vi "ReadEncoders.vi"(0 "Reset Encoders":bool, 5 "Cluster in":T1={FALSE, "Tick Count(uSec)"=0, "Counter Value"=[0, 0, 0, 0], "x-y"=[0, 0, 0, 0]}, 11 "error in (no error)":errorcluster) -> (4 "Tick Count(uSec)":u32 caption="Tick Count(Ticks)", 8 "output cluster":T2, 13 "Cluster Out":T1, 14 "Updated":bool, 15 "error out":errorcluster)   [LabVIEW 2018]
uses:
  <vilib>/myRIO/Common/Instrument Driver Framework/myRIO v1.0/Encoder/typedefs/Encoder Signal Mode.ctl
  <vilib>/myRIO/Instrument Drivers/Onboard IO/Encoder/typedefs/Encoder Reference.ctl
  <vilib>/myRIO/Common/Instrument Driver Framework/Utilities/typedefs/myRIO Generic Hardware Reference.ctl
  <vilib>/myRIO/Common/Instrument Driver Framework/Utilities/typedefs/Hardware Version Enum.ctl
  <vilib>/myRIO/Common/Instrument Driver Framework/Utilities/typedefs/myRIO v1.0 Reference.ctl
  <vilib>/myRIO/Common/Instrument Driver Framework/Utilities/typedefs/Generic FPGA Reference.ctl
  <vilib>/myRIO/Common/Instrument Driver Framework/myRIO v1.0/Encoder/typedefs/Encoder Channels Enum.ctl
  <vilib>/myRIO/Common/Instrument Driver Framework/myRIO v1.0/Encoder/typedefs/Encoder Configuration v1.0.ctl
  <vilib>/userdefined/High Color/nirio_resource_hc.ctl
  <vilib>/myRIO/Common/Instrument Driver Framework/Utilities/vis/Is FPGA Ref Available.vi
  <vilib>/myRIO/Common/Instrument Driver Framework/myRIO v1.0/Encoder/vis/myRIO v1.1 Open Encoder.vi
  <vilib>/myRIO/Instrument Drivers/Onboard IO/Encoder/vis/Read.vi
  <vilib>/myRIO/Common/Instrument Driver Framework/Utilities/vis/Validate Channels.vi
  <vilib>/myRIO/Common/Instrument Driver Framework/myRIO v1.0/Encoder/vis/myRIO v1.0 Reserve Encoder.vi
  <vilib>/myRIO/Common/Instrument Driver Framework/myRIO v1.0/Encoder/vis/myRIO v1.0 Build MUX Configuration Encoder.vi
  <vilib>/myRIO/Common/Instrument Driver Framework/myRIO v1.0/Resource Manager/vis/myRIO v1.0 Reserve Channel List.vi
  <vilib>/myRIO/Common/Instrument Driver Framework/myRIO v1.0/Resource Manager/vis/myRIO v1.0 Create Configuration List.vi
  <vilib>/myRIO/Common/Instrument Driver Framework/myRIO v1.0/Resource Manager/vis/myRIO v1.0 Reserve Channel.vi
  <vilib>/myRIO/Common/Instrument Driver Framework/myRIO v1.0/Resource Manager/vis/myRIO v1.0 Unreserve Channel.vi
  <vilib>/myRIO/Common/Instrument Driver Framework/myRIO v1.0/Resource Manager/vis/myRIO v1.0 Build Mutex Name.vi
  <vilib>/Utility/VariantDataType/GetNumericInfo.vi
  <vilib>/Utility/error.llb/Error Cluster From Error Code.vi
  <vilib>/myRIO/Common/Instrument Driver Framework/myRIO v1.0/myRIO v1.1 Open.vi
  <vilib>/myRIO/Common/Instrument Driver Framework/Utilities/vis/IO Manager.vi
  <vilib>/myRIO/Common/Instrument Driver Framework/Utilities/vis/Configuration Manager.vi
  <vilib>/myRIO/Common/Instrument Driver Framework/myRIO v1.0/Resource Manager/vis/myRIO v1.0 Configure IO.vi
  <vilib>/myRIO/Common/Instrument Driver Framework/myRIO v1.0/myRIO v1.0 Close.vi
  <vilib>/myRIO/Common/Instrument Driver Framework/myRIO v1.0/Encoder/vis/myRIO v1.0 Configure Encoder.vi
  <vilib>/myRIO/Common/Instrument Driver Framework/myRIO v1.0/Encoder/vis/myRIO v1.0 Read Encoder.vi
  <vilib>/myRIO/Express VI/Onboard IO/Encoder/Encoder Express VI.xnode
  <vilib>/myRIO/Instrument Drivers/Onboard IO/Encoder/vis/myRIO Encoder Open.xnode
  <vilib>/myRIO/Common/Instrument Driver Framework/myRIO v1.0/Encoder/typedefs/Encoder Count Direction Enum.ctl
  <vilib>/rvi/Arithmetic/AddSubMult/XNode/nirviSatArithmetic.xnode
  <vilib>/myRIO/Instrument Drivers/Onboard IO/Encoder/Encoder.lvlib
panel:
  out "CM Oikea":dbl
  out "CM Vasen":dbl
  out "CM Etu":dbl
  out "CM Taka":dbl
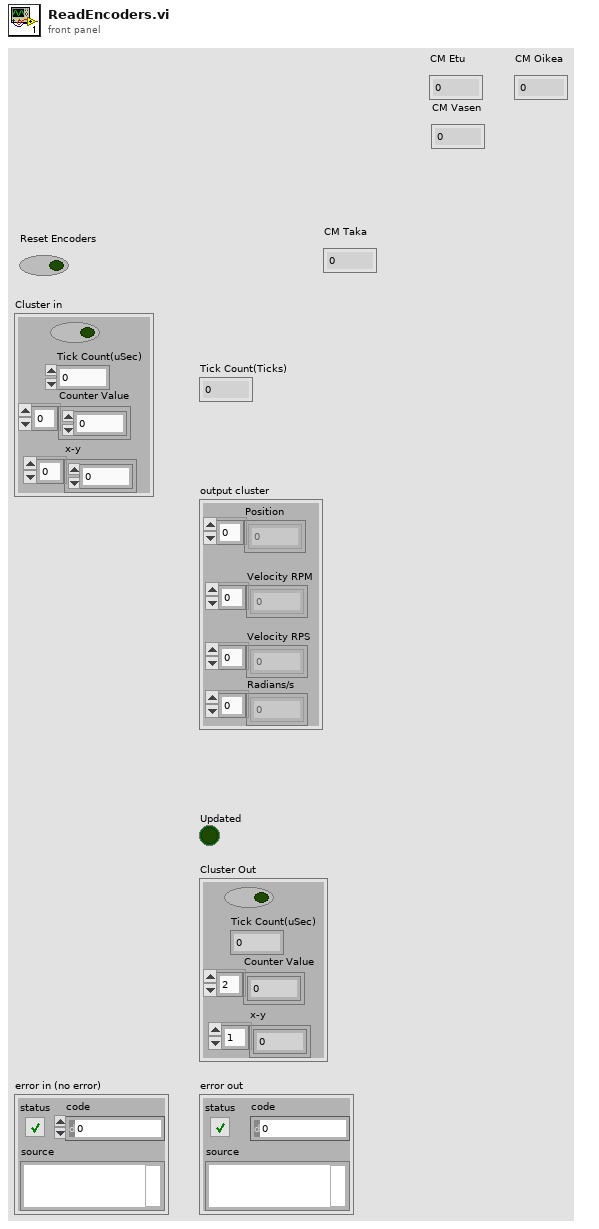
[diagram p1: front panel]
types:
  T1 = cluster{bool, "Tick Count(uSec)":u32, "Counter Value":i32[], "x-y":i32[]}
  T2 = cluster{"Position":i32[], "Velocity RPM":dbl[], "Velocity RPS":dbl[], "Radians/s":dbl[]}
  T3 = cluster{"Counter Value":i32[], dbl[], dbl[], dbl[]}
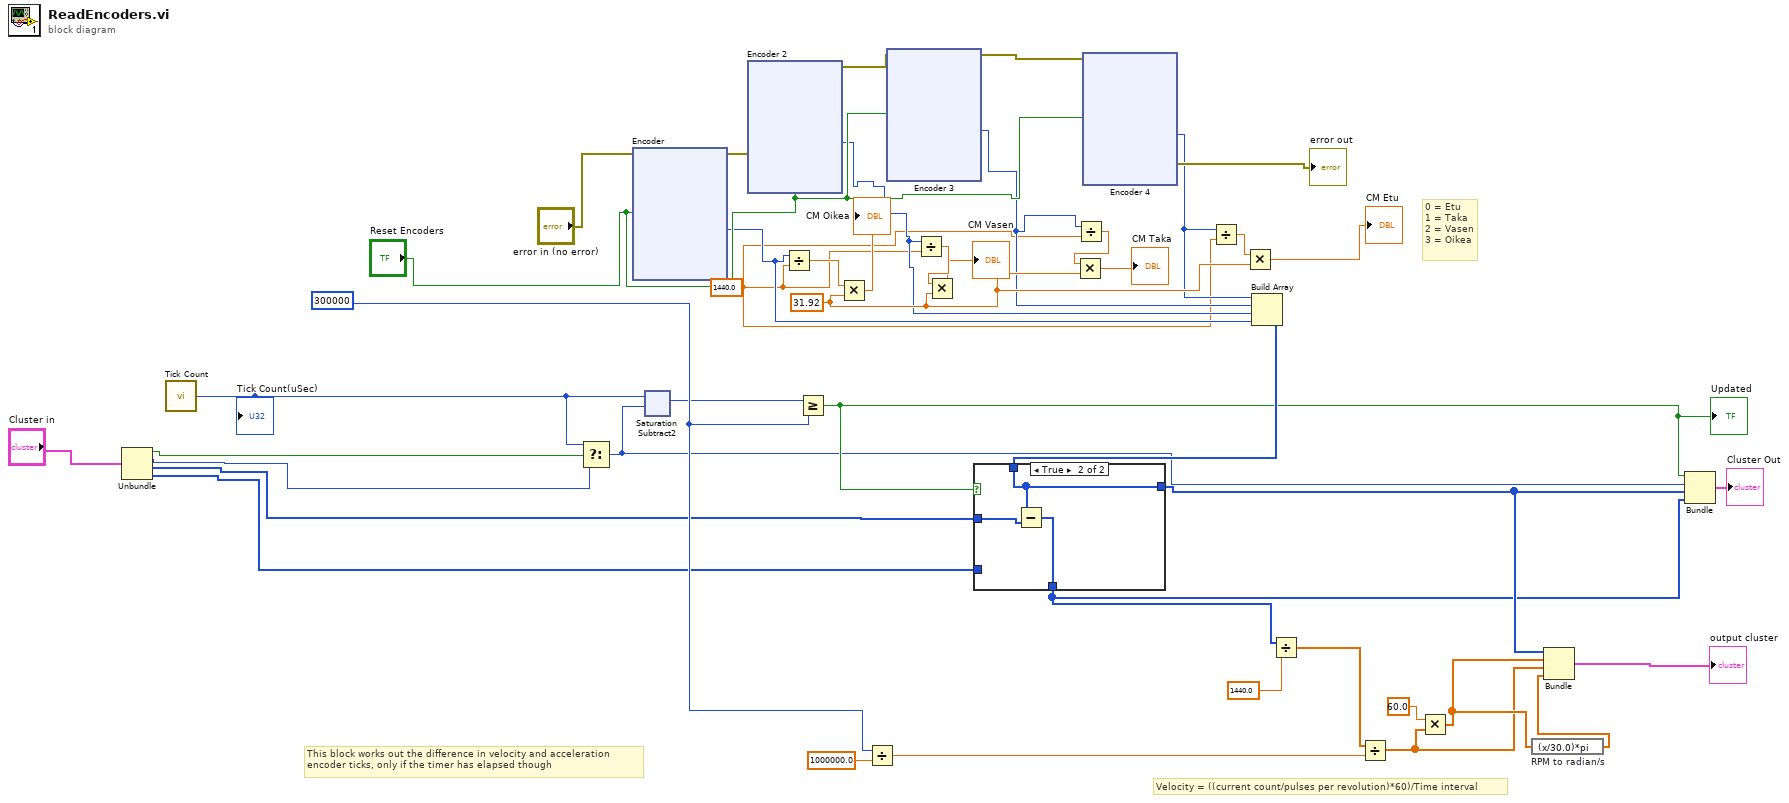
[diagram p0: block diagram]
diagram:
  w2 = 1440.0
  w11 = 31.92
  w42 = 300000
  # "0 = Etu\n1 = Taka\n2 = Vasen\n3 = Oikea"
  # "Velocity = ((current count/pulses per revolution)*60)/Time interval"
  # "This block works out the difference in velocity and acceleration \nencoder ticks, only if the timer has elapsed though"
  n1 = Unbundle("Cluster in") -> (w32:bool, "Tick Count(uSec)"=w33:u32, "Counter Value"=w34:i32[], "x-y"=w35:i32[])
  n2 = call "Tick Count"() -> ("Tick Count(uSec)"=w22:u32)
  "Tick Count(uSec)" <- w22
  n3 = Select(t=w22, s=w32, f=w33) -> (s? t:f=w23:u32)
  n4 = xnode "Encoder"("Reset Counter"="Reset Encoders", "error in (no error)"="error in (no error)") -> ("Counter Value"=w14:i32, "error out"=w28:errorcluster)  [unwired: 2 out]
  n5 = xnode ("Saturation Subtract2")("x"=w22, "y"=w23) -> ("x-y"=w27:u32)
  n6 = xnode "Encoder 2"("Reset Counter"="Reset Encoders", "error in (no error)"=w28) -> ("Counter Value"=w6:i32, "error out"=w39:errorcluster)  [unwired: 2 out]
  n7 = Divide(x=w14, y=w2) -> (x/y=w13:dbl)
  n8 = Greater Or Equal?(x=w27, y=w42) -> (x >= y?=w24:bool)
  "Updated" <- w24
  n9 = Multiply(x=w13, y=w11) -> (x*y=→"CM Oikea":dbl)
  n10 = Divide(x=w42, y=1000000.0) -> (x/y=w20:dbl)
  n11 = xnode "Encoder 3"("Reset Counter"="Reset Encoders", "error in (no error)"=w39) -> ("Counter Value"=w5:i32, "error out"=w40:errorcluster)  [unwired: 2 out]
  n12 = Divide(x=w6, y=w2) -> (x/y=w7:dbl)
  n13 = Multiply(x=w7, y=w11) -> (x*y=→"CM Vasen":dbl)
  n14 = Divide(x=w5, y=w2) -> (x/y=w8:dbl)
  n15 = Multiply(x=w8, y=w11) -> (x*y=→"CM Taka":dbl)
  n16 = xnode "Encoder 4"("Reset Counter"="Reset Encoders", "error in (no error)"=w40) -> ("Counter Value"=w3:i32, "error out"=→"error out":errorcluster)  [unwired: 2 out]
  n17 = Divide(x=w3, y=w2) -> (x/y=w9:dbl)
  n18 = Multiply(x=w9, y=w11) -> (x*y=→"CM Etu":dbl)
  n19 = Build Array(w3, w5, w6, w14) -> (w29:i32[])
  n20 = case shown="True" w24 {
    tunnel: w34 -> [w44 w48]
    tunnel: [w45 w47] -> w19
    tunnel: w35 -> [w45 _]
    tunnel: [w44 w46] -> w21
    tunnel: w29 -> [_ w46]
    frame False {
    }
    frame True {
      n21 = Subtract(x=w46, y=w48) -> (x-y=w47:i32[])
    }
  }
  n22 = Divide(x=w19, y=1440.0) -> (x/y=w18:dbl[])
  n23 = Divide(x=w18, y=w20) -> (x/y=w17:dbl[])
  n24 = Multiply(x=60.0 ("y"), y=w17) -> (x*y=w36:dbl[])
  n25 = expression code="(x/30.0)*pi" "RPM to radian/s"(w36) -> (w37:dbl[])
  n26 = Bundle("Counter Value"=w21, w36, w17, w37) -> (→"output cluster":T3)  [unwired: 1 in]
  n27 = Bundle(w24, "Tick Count(uSec)"=w23, "Counter Value"=w21, "x-y"=w19) -> (→"Cluster Out":T1)  [unwired: 1 in]
